vi "Interpret System Message Event Data.vi"(8 "Sys. Msg. Origin":string, 9 "Sys. Msg. Source":T1, 10 "Payload":variant, 11 "Identifier":string) -> (0 "error out":errorcluster, 1 "Additional Info":string, 2 "Module ID":i32, 3 "Module Name":string)   [LabVIEW 2022 SP3, in "Event Manager.lvlib"]
doc: "____\nHAMPEL SOFTWARE ENGINEERING v2.6.0 (2023-12-19 10:54)"
uses:
  Event Manager.lvlib
  Libraries/hse-libraries/Source/hse-dqmh/Controls/System Message Source.ctl
  Libraries/hse-libraries/Source/hse-dqmh/Controls/System Message - Add to Run-Time Menu - Argument--cluster.ctl
  Libraries/hse-libraries/Source/hse-dqmh/Controls/System Message Framework Identifiers.ctl
  Libraries/hse-libraries/Source/hse-dqmh/Controls/System Message - Removed from Subpanel - Payload--cluster.ctl
  Libraries/hse-libraries/Source/hse-dqmh/Controls/System Message - Ready for Display - Payload--cluster.ctl
  Libraries/hse-libraries/Source/hse-dqmh/hse-dqmh.lvlib
panel:
  in  "error in":errorcluster
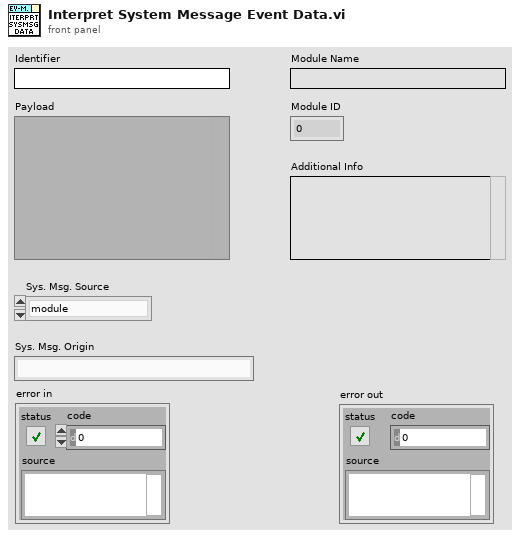
[diagram p1: front panel]
types:
  T1 = typedef "hse-dqmh.lvlib/System Message Source.ctl" = enum16{"module", "application", "network"}
  T2 = typedef "hse-dqmh.lvlib/System Message - Add to Run-Time Menu - Argument--cluster.ctl" = cluster{"Module Disk Path":path, "Module Descriptor":string}
  T3 = typedef "hse-dqmh.lvlib/System Message Framework Identifiers.ctl" = enum16{"Add to Run-Time Menu", "Ready for Display", "Removed from Subpanel", "Remove from Run-Time Menu"}
  T4 = typedef "hse-dqmh.lvlib/System Message - Removed from Subpanel - Payload--cluster.ctl" = cluster{"Removed Module":string}
  T5 = typedef "hse-dqmh.lvlib/System Message - Ready for Display - Payload--cluster.ctl" = cluster{"Module Path":path, "VI Reference":refnum<vi>, "Title":string, "Target SP Name":string}
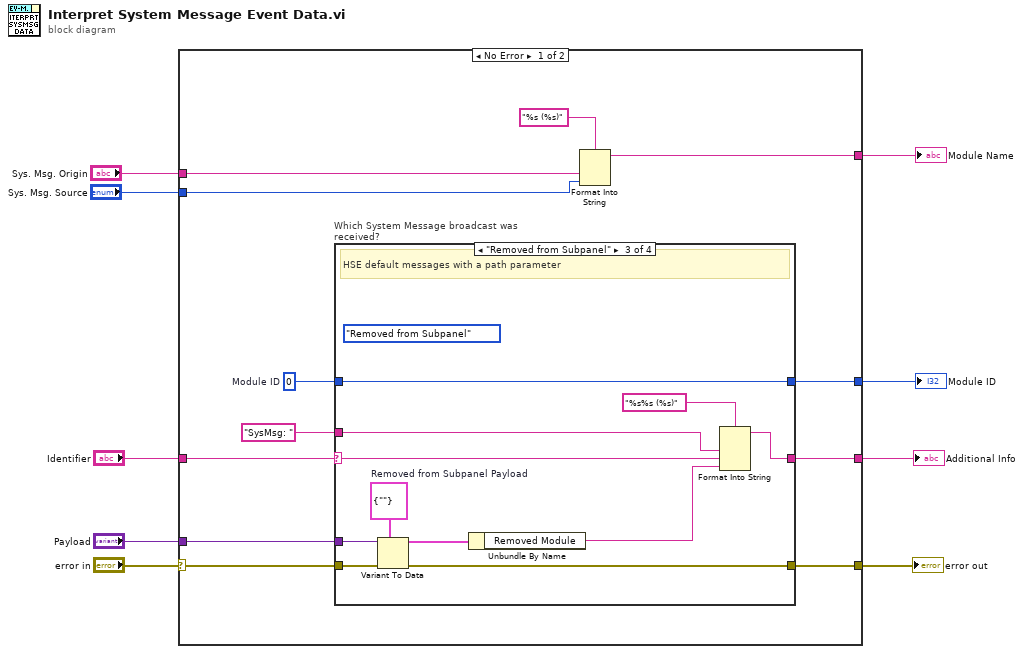
[diagram p0: block diagram]
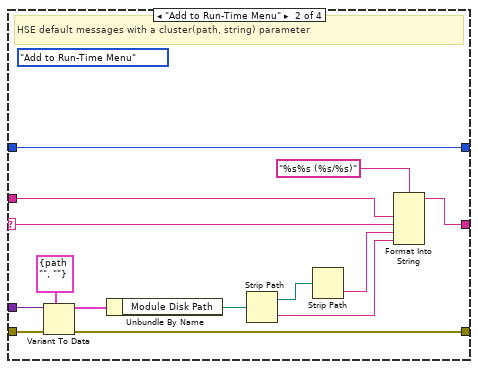
[diagram p3: hidden frame]
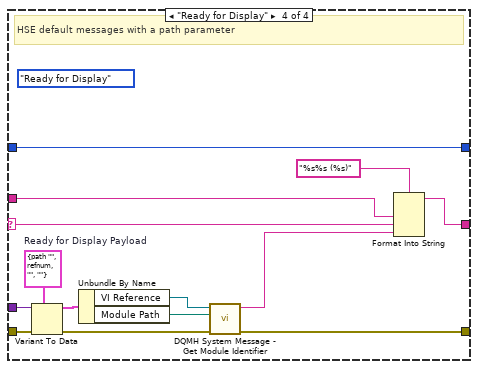
[diagram p4: hidden frame]
diagram:
  n1 = case shown="No Error" "error in" {
    selector: "error in" -> [w11 w64]
    tunnel: "Identifier" -> [w21 _]
    tunnel: "Sys. Msg. Source" -> [w20 _]
    tunnel: [w19 _] -> w7
    tunnel: "Payload" -> [w17 _]
    tunnel: [w16 _] -> w5
    tunnel: [w15 _] -> w4
    tunnel: "Sys. Msg. Origin" -> [w14 _]
    tunnel: [w10 w64] -> w1
    frame No Error {
      w13 = 0  # Module ID
      n2 = case "Which System Message broadcast was received?" shown="\"Removed from Subpanel\"" w21 {
        selector: w21 -> [w24 w37 w48 w62]
        tunnel: w17 -> [_ w36 w47 w56]
        tunnel: [w24 w35 w46 w61] -> w16
        tunnel: [w23 w34 w45 w60] -> w15
        tunnel: w13 -> [w23 w34 w45 w60]
        tunnel: "SysMsg: " ("format string") -> [_ w29 w44 w59]
        tunnel: [w22 w25 w43 w53] -> w10
        tunnel: w11 -> [w22 w26 w42 w55]
        frame Default {
          # "Anything else..."
        }
        frame "Add to Run-Time Menu" {
          (unwired) System_Message_Framework_Identifiers."Add to Run-Time Menu" ("System Message Identifiers")
          # "HSE default messages with a cluster(path, string) parameter"
          n3 = Variant To Data(error in=w26, type=T2 {"Module Disk Path"=path "", "Module Descriptor"=""} ("Add to RTM Argument"), Variant=w36) -> (data=w33:T2, error out=w25:errorcluster)
          n4 = Unbundle By Name(w33) -> ("Module Disk Path"=w27:path)
          n5 = Strip Path(path=w27) -> (stripped path=w32:path, name=w30:string)
          n6 = Strip Path(path=w32) -> (name=w31:string)  [unwired: 1 out]
          n7 = Format Into String(format string="%s%s (%s/%s)", w29, w37, w31, w30) -> (resulting string=w35:string)  [unwired: 2 in, 1 out]
        }
        frame "Removed from Subpanel" {
          w41 = T4 {"Removed Module"=""}  # Removed from Subpanel Payload
          (unwired) System_Message_Framework_Identifiers."Removed from Subpanel" ("System Message Identifiers")
          # "HSE default messages with a path parameter"
          n8 = Variant To Data(error in=w42, type=w41, Variant=w47) -> (data=w40:T4, error out=w43:errorcluster)
          n9 = Unbundle By Name(w40) -> ("Removed Module"=w39:string)
          n10 = Format Into String(format string="%s%s (%s)", w44, w48, w39) -> (resulting string=w46:string)  [unwired: 2 in, 1 out]
        }
        frame "Ready for Display" {
          w57 = T5 {"Module Path"=path "", "VI Reference"=refnum, "Title"="", "Target SP Name"=""}  # Ready for Display Payload
          (unwired) System_Message_Framework_Identifiers."Ready for Display" ("System Message Identifiers")
          # "HSE default messages with a path parameter"
          n11 = Variant To Data(error in=w55, type=w57, Variant=w56) -> (data=w58:T5, error out=w54:errorcluster)
          n12 = Unbundle By Name(w58) -> ("VI Reference"=w51:refnum<vi>, "Module Path"=w52:path)
          n13 = call "DQMH System Message - Get Module Identifier.vi"("error in (no error)"=w54, "Module Path"=w52, "VI Ref"=w51) -> ("error out"=w53:errorcluster, "Module Identifier"=w50:string)  [unwired: 7 in]
          n14 = Format Into String(format string="%s%s (%s)", w59, w62, w50) -> (resulting string=w61:string)  [unwired: 2 in, 1 out]
        }
      }
      n15 = Format Into String(format string="%s (%s)", w14, w20) -> (resulting string=w19:string)  [unwired: 2 in, 1 out]
    }
    frame Error {
    }
  }
  "Additional Info" <- w5
  "Module Name" <- w7
  "Module ID" <- w4
  "error out" <- w1
